vi "midioutopen.vi"(4 "error in (no error)":errorcluster, 7 "uDeviceID":u32) -> (0 "error out":errorcluster, 2 "Win32 Error Code":i32, 3 "hmidiout handle":i32)   [LabVIEW 2014]
doc: "Opens a reference to a MIDI Output Device."
uses:
  winmm.dll
panel:
  # "Input Data"
  # "Local Data"
  # "Output Data"
  # "No local data."
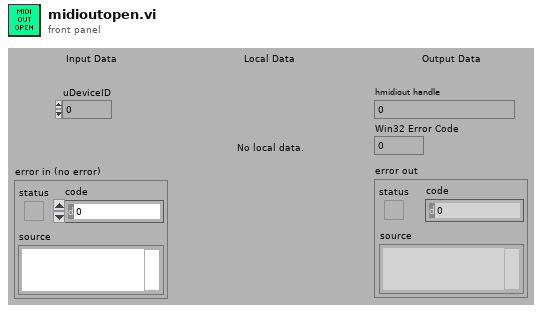
[diagram p1: front panel]
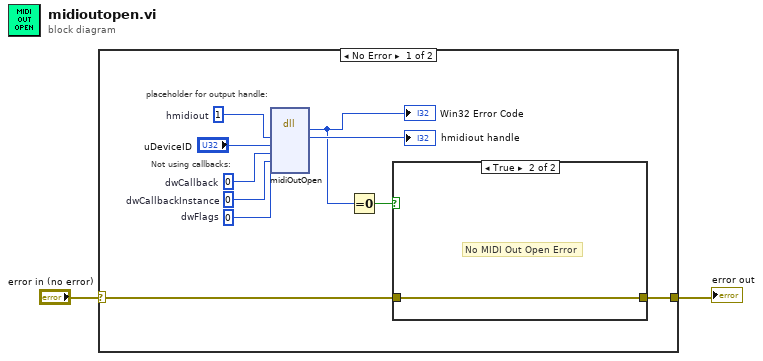
[diagram p0: block diagram]
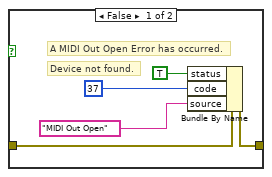
[diagram p2: hidden frame]
diagram:
  n1 = case shown="No Error" "error in (no error)" {
    selector: "error in (no error)" -> [w5 w19]
    tunnel: [w4 w19] -> w1
    frame No Error {
      w7 = 0  # dwFlags
      w8 = 0  # dwCallbackInstance
      w9 = 0  # dwCallback
      w11 = 1  # hmidiout
      # "placeholder for output handle:"
      # "Not using callbacks:"
      n2 = dll-call lib="winmm.dll" fn="midiOutOpen"("hmidiout"=w11, "uDeviceID"="uDeviceID", "dwCallback"=w9, "dwCallbackInstance"=w8, "dwFlags"=w7) -> (w3:i32, "hmidiout"=→"hmidiout handle":i32)  [unwired: 7 in, 2 out]
      "Win32 Error Code" <- w3
      n3 = Equal To 0?(x=w3) -> (x = 0?=w6:bool)
      n4 = case shown="True" w6 {
        tunnel: w5 -> [w16 w18]
        tunnel: [w15 w18] -> w4
        frame False {
          # "Device not found."
          # "A MIDI Out Open Error has occurred."
          n5 = Bundle By Name(cluster=w16, "status"=TRUE ("element"), "code"=37, "source"="MIDI Out Open") -> (w15:errorcluster)
        }
        frame True {
          # "No MIDI Out Open Error"
        }
      }
    }
    frame Error {
    }
  }
  "error out" <- w1
